vi "Commit Build Settings.vi"(8 "error in (no error)":errorcluster, 11 "SDIST in":refnum<class "NI_AB_API_SDIST.lvclass">) -> (0 "error out":errorcluster, 3 "SDIST out":refnum<class "NI_AB_API_SDIST.lvclass">)   [LabVIEW 2020, in "NI_AB_API_SDIST.lvclass"]
uses:
  <vilib>/AppBuilder/AB_API/SDIST/NI_AB_API_SDIST.lvclass
  <vilib>/AppBuilder/AB_API/SDIST/NI_AB_API_SDIST.lvclass/NI_AB_API_SDIST.ctl
  <vilib>/AppBuilder/AB_API/Build/NI_AB_API_Build.lvclass
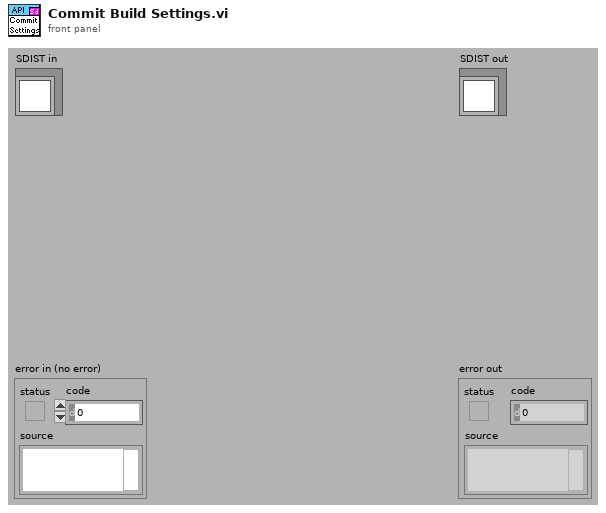
[diagram p1: front panel]
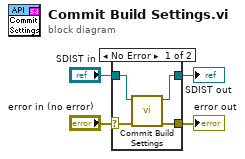
[diagram p0: block diagram]
diagram:
  n1 = case shown="No Error" "error in (no error)" {
    selector: "error in (no error)" -> [w6 w10]
    tunnel: [w5 w10] -> w3
    tunnel: [w7 w9] -> w1
    tunnel: "SDIST in" -> [w8 w9]
    frame No Error {
      n2 = call-parent "Commit Build Settings.vi"("error in (no error)"=w6, "Build in"=w8) -> ("error out"=w5:errorcluster, "Build out"=w7:refnum<class "NI_AB_API_SDIST.lvclass">)  [unwired: 8 in]
    }
    frame Error {
    }
  }
  "error out" <- w3
  "SDIST out" <- w1
